vi "NameOrGUID.vi"(0 "Name":string) -> (14 "NameOrGUID":string)   [LabVIEW 2019, in "Error handler.lvclass"]
uses:
  Error handler.lvclass
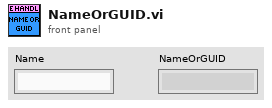
[diagram p1: front panel]
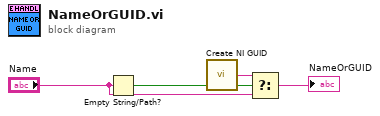
[diagram p0: block diagram]
diagram:
  n1 = Empty String/Path?(string/path="Name") -> (empty?=w4:bool)
  n2 = call <vilib>:"Create NI GUID.vi"() -> ("NI GUID"=w1:string)
  n3 = Select(t=w1, s=w4, f="Name") -> (s? t:f=→"NameOrGUID":string)
